vi "projeee hakan.vi"() -> ()   [LabVIEW 2018]
uses:
  <vilib>/LabVIEW Interface for Arduino/Type Defs/Board Type.ctl
  <vilib>/LabVIEW Interface for Arduino/Type Defs/Pin Mode.ctl
  <vilib>/LabVIEW Interface for Arduino/LabVIEW Interface for Arduino.lvlib
panel:
  in  "stop 2":bool
  in  "file path (use dialog)":path
  in  "stop":bool
  out "ölçülen sıcaklık değeri":dbl(knob) scale=0.0..100.0
  in  "VISA resource":refnum<visa-resource-name>
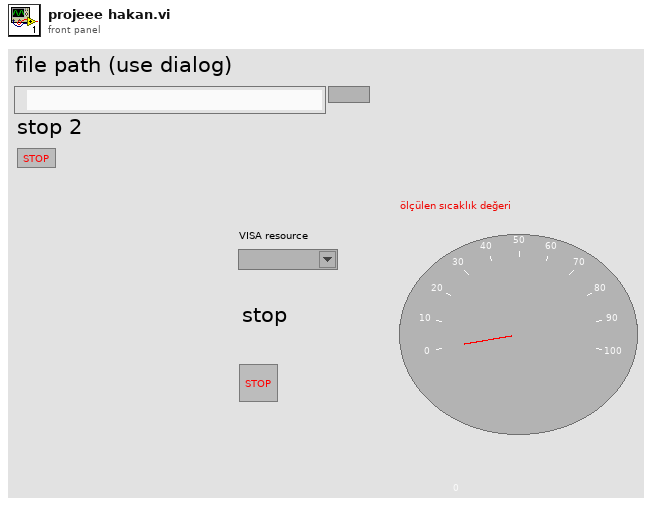
[diagram p1: front panel]
types:
  T1 = enum16{"open", "replace", "create", "open or create", "replace or create", "replace or create with confirmation"}
  T2 = typedef "LabVIEW Interface for Arduino.lvlib/Board Type.ctl" = enum16{"Uno", "Dimuelanove w/Atmega 328", "Mega 2560"}
  T3 = typedef "LabVIEW Interface for Arduino.lvlib/Arduino Resource.ctl" = cluster{"VISA resource":refnum<visa-resource-name>, "Board Type":T2, "Connection Type":enum8{"USB / Serial"}, "Bytes Per Packet (15)":u8}
  T4 = typedef "LabVIEW Interface for Arduino.lvlib/Pin Mode.ctl" = enum8{"Input", "Output"}
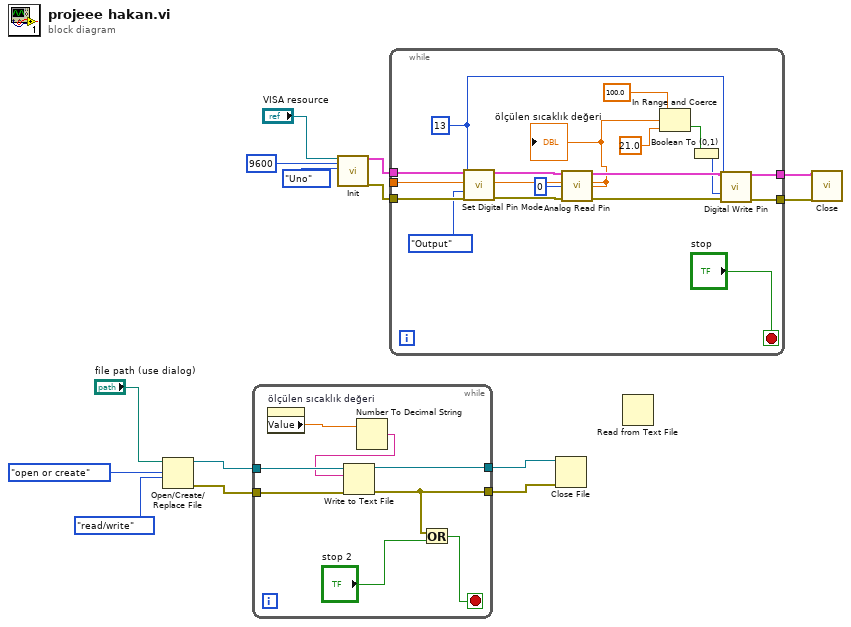
[diagram p0: block diagram]
diagram:
  n1 = Open/Create/Replace File(file path (use dialog)="file path (use dialog)", operation (0:open)=T1."open or create", access (0:read/write)=enum16{"read/write", "read-only", "write-only"}."read/write") -> (refnum out=w4:refnum<file>, error out=w2:errorcluster)  [unwired: 3 in, 1 out]
  n2 = while {
    tunnel: w4 -> [w22]
    tunnel: [w21] -> w3
    tunnel: w2 -> [w20]
    tunnel: [w18] -> w1
    stop <- w17 stop-if-true
    n3 = property on="ölçülen sıcaklık değeri" class="Knob (strict)"() -> ("Value"=w16:dbl)  [unwired: 2 in, 2 out]
    n4 = Number To Decimal String(number=w16) -> (decimal integer string=w15:string)  [unwired: 1 in]
    n5 = Write to Text File(file (use dialog)=w22, text=w15, error in=w20) -> (refnum out=w21:refnum<file>, error out=w18:errorcluster)  [unwired: 1 in, 1 out]
    n6 = Or(x=w18, y="stop 2") -> (x .or. y?=w17:bool)
  }
  n7 = call <vilib>:"Init.vi"("VISA resource"="VISA resource", "Baud Rate (115200)"=u32 9600, "Board Type (Uno)"=Board_Type."Uno") -> ("Arduino Resource"=w11:T3, "error out"=w10:errorcluster)  [unwired: 15 in]
  n8 = while {
    tunnel: w11 -> [w39]
    tunnel: w10 -> [w38]
    tunnel: [w28] -> w9
    tunnel: [w27] -> w8
    tunnel: [w23] -> _
    stop <- "stop" stop-if-true
    w25 = u8 13 ("Digital I/O Pin")
    n9 = call <vilib>:"Set Digital Pin Mode.vi"("Arduino Resource"=w39, "Digital I/O Pin"=w25, "Pin Mode (Input)"=Pin_Mode."Output", "error in"=w38) -> ("Arduino Resource"=w36:T3, "error out"=w34:errorcluster)  [unwired: 10 in]
    n10 = call <vilib>:"Analog Read Pin.vi"("Arduino Resource"=w36, "Analog Input Pin (0)"=u8 0, "error in"=w34) -> ("Arduino Resource"=w30:T3, "Voltage"=w23:dbl, "error out"=w29:errorcluster)  [unwired: 10 in]
    "ölçülen sıcaklık değeri" <- w23
    n11 = In Range and Coerce(upper limit=100.0, x=w23, lower limit=21.0) -> (In Range?=w31:bool)  [unwired: 1 out]
    n12 = Boolean To (0,1)(Boolean=w31) -> (0, 1=w24:i16)
    n13 = call <vilib>:"Digital Write Pin.vi"("Arduino Resource"=w30, "Digital I/O Pin (0)"=w25, "Value (0)"=w24, "error in"=w29) -> ("Arduino Resource"=w28:T3, "error out"=w27:errorcluster)  [unwired: 10 in]
  }
  n14 = Close File(refnum=w3, error in=w1) -> ()  [unwired: 2 out]
  n15 = Read from Text File() -> ()  [unwired: 4 in, 4 out]
  n16 = call <vilib>:"Close.vi"("Arduino Resource"=w9, "error in"=w8) -> ()  [unwired: 13 in, 1 out]
